vi "Set Initialization Data - Status Platine Newport.vi"(8 "error in":errorcluster, 11 "UI SmarAct in":refnum<class "UI SmarAct.lvclass">) -> (0 "error out":errorcluster, 3 "UI SmarAct out":refnum<class "UI SmarAct.lvclass">)   [LabVIEW 2024, in "UI SmarAct.lvclass"]
doc: "In this VI you can set the initialization data of a statically-linked subWorker."
uses:
  UI SmarAct.lvclass
  C:/Program Files (x86)/National Instruments/LabVIEW 2024/vi.lib/addons/_Workers/Library/Classes/Worker/Worker.lvclass
  Status Platine Newport/Initialization Data.ctl
  Status Platine Newport/Response Cases.ctl
  UI SmarAct.lvclass/UI SmarAct.ctl
  Status Platine Newport/Status Platine Newport.lvclass
  C:/Program Files (x86)/National Instruments/LabVIEW 2024/vi.lib/addons/_Workers/Library/Classes/Workers Object/Workers Object.lvclass
  C:/Users/flepetit/Desktop/FROG-SHG-LV2024/Workers/Status Platine Newport/Status Platine Newport.lvclass
  Newport.SMC100.CommandInterface
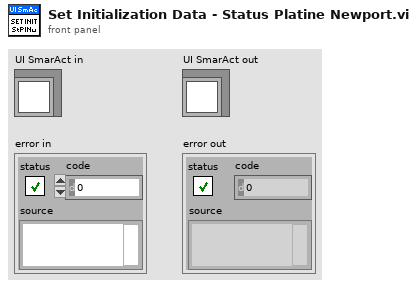
[diagram p1: front panel]
types:
  T1 = typedef "Status Platine Newport.lvclass/Initialization Data.ctl" = cluster{"Response Cases":T2}
  T2 = typedef "Status Platine Newport.lvclass/Response Cases.ctl" = cluster{"Placeholder - Can be deleted":string, "SMC100 Reference":refnum<k24>, "RefnumStatus Platine":refnum<vi>}
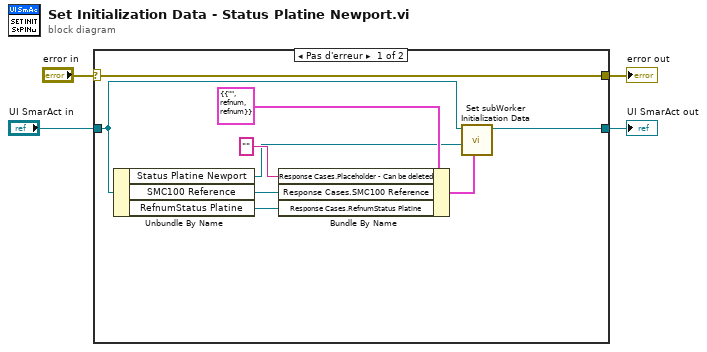
[diagram p0: block diagram]
diagram:
  n1 = case shown="Pas d'erreur" "error in" {
    selector: "error in" -> [w13 w15]
    tunnel: [w13 w15] -> w2
    tunnel: [w12 w14] -> w1
    tunnel: "UI SmarAct in" -> [w11 w14]
    frame No Error {
      n2 = Unbundle By Name(w11) -> ("Status Platine Newport"=w5:refnum<class "Status Platine Newport.lvclass">, "SMC100 Reference"=w7:refnum<k24>, "RefnumStatus Platine"=w6:refnum<vi>)
      n3 = Bundle By Name(cluster=T1 {"Response Cases"={"Placeholder - Can be deleted"="", "SMC100 Reference"=refnum, "RefnumStatus Platine"=refnum}} ("Initialization Data"), "Response Cases.Placeholder - Can be deleted"="" ("Placeholder"), "Response Cases.SMC100 Reference"=w7, "Response Cases.RefnumStatus Platine"=w6) -> (w9:T1)
      n4 = call-dynamic "Set subWorker Initialization Data.vi"("Initialization Data"=w9, "subWorker"=w5, "Worker"=w11) -> ("Worker out"=w12:refnum<class "UI SmarAct.lvclass">)  [unwired: 8 in]
    }
    frame Error {
    }
  }
  "error out" <- w2
  "UI SmarAct out" <- w1
